vi "Мультиплексор 1.vi"(0 "1":T2, 1 "2":T2, 2 "3":T2, 3 "4":T2, 4 "adrA":cluster{"Boolean":bool, "Boolean 2":bool}) -> (5 "Cluster":T1)   [LabVIEW 2017]
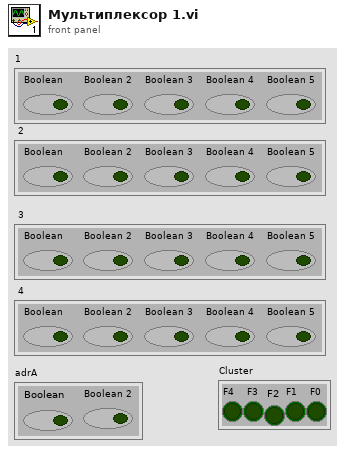
[diagram p1: front panel]
types:
  T1 = cluster{"F4":bool, " F3":bool, "F2":bool, "F1":bool, " F0":bool}
  T2 = cluster{"Boolean":bool, "Boolean 2":bool, "Boolean 3":bool, "Boolean 4":bool, "Boolean 5":bool}
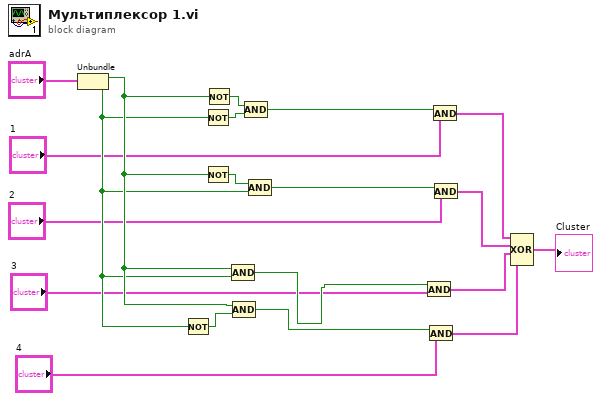
[diagram p0: block diagram]
diagram:
  n1 = Unbundle("adrA") -> ("Boolean"=w15:bool, "Boolean 2"=w14:bool)
  n2 = Not(x=w14) -> (.not. x?=w20:bool)
  n3 = Not(x=w14) -> (.not. x?=w17:bool)
  n4 = Not(x=w15) -> (.not. x?=w19:bool)
  n5 = Not(x=w15) -> (.not. x?=w18:bool)
  n6 = Compound Arithmetic op=AND(w15, w14) -> (w11:bool)
  n7 = Compound Arithmetic op=AND(w15, w20) -> (w10:bool)
  n8 = Compound Arithmetic op=AND(w18, w17) -> (w12:bool)
  n9 = Compound Arithmetic op=AND(w19, w14) -> (w13:bool)
  n10 = And(x=w11, y="3") -> (x .and. y?=w3:T2)
  n11 = And(x=w10, y="4") -> (x .and. y?=w2:T2)
  n12 = And(x=w12, y="1") -> (x .and. y?=w5:T2)
  n13 = And(x=w13, y="2") -> (x .and. y?=w4:T2)
  n14 = Compound Arithmetic op=XOR(w5, w4, w3, w2) -> (→"Cluster":T2)
